vi "ReadParameters.vi"(8 "error in (no error)":errorcluster, 11 "Step in":refnum<class "Step.lvclass">) -> (0 "error out":errorcluster, 2 "Parameters":refnum<class "Parameter.lvclass">[](array[class]), 3 "Step out":refnum<class "Step.lvclass">)   [LabVIEW 2023, in "Easy.SequenceManagerLabVIEW.lvlib" / "Step.lvclass"]
uses:
  Step.lvclass
  Step.lvclass/Step.ctl
  Parameter/Parameter.lvclass
panel:
  # "Connector Pane"
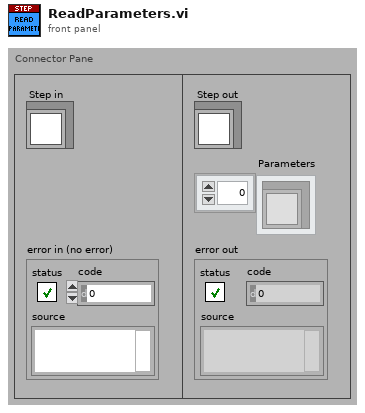
[diagram p1: front panel]
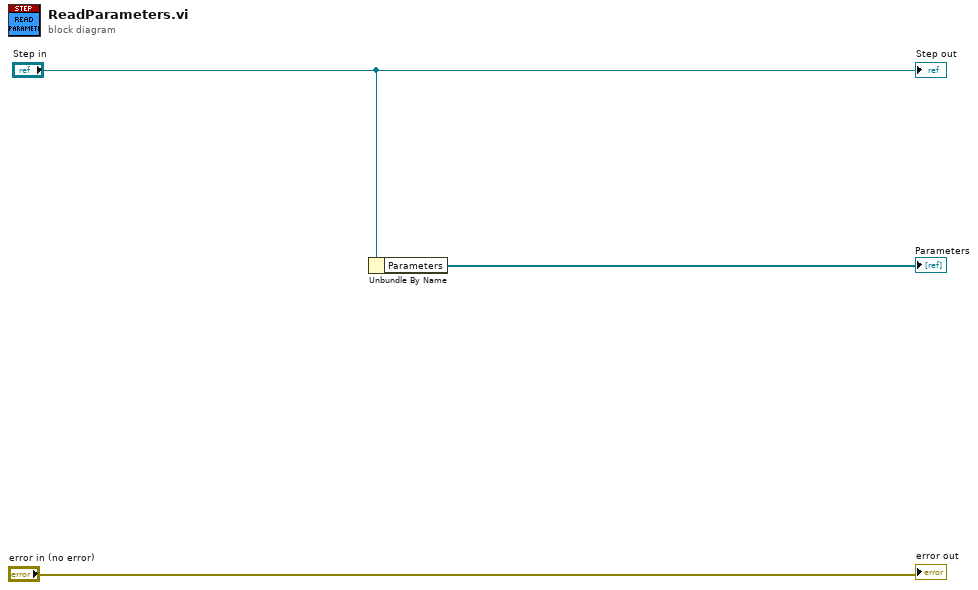
[diagram p0: block diagram]
diagram:
  n1 = Unbundle By Name("Step in") -> ("Parameters"=→"Parameters":refnum<class "Parameter.lvclass">[])
  "error out" <- "error in (no error)"
  "Step out" <- "Step in"
